vi "AddPerformancePropertiesToWaveform.vi"(6 "Waveform":waveform(sgl), 8 "error in (no error)":errorcluster, 9 "Channel":string, 10 "Group":string, 11 "Tdms Ref":refnum<k34>) -> (0 "error out":errorcluster, 1 "Channel out":string, 2 "Group out":string, 3 "Tdms Ref out":refnum<k34>)   [LabVIEW 2017, in "DataExplorerSupport.lvlib"]
uses:
  <vilib>/addons/InsightCM/Utilities/DataExplorerSupport/DataExplorerSupport.lvlib
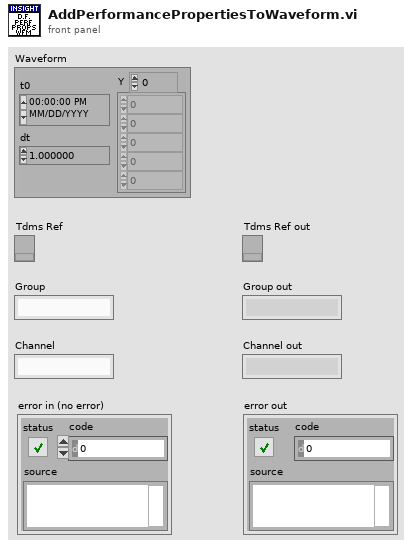
[diagram p1: front panel]
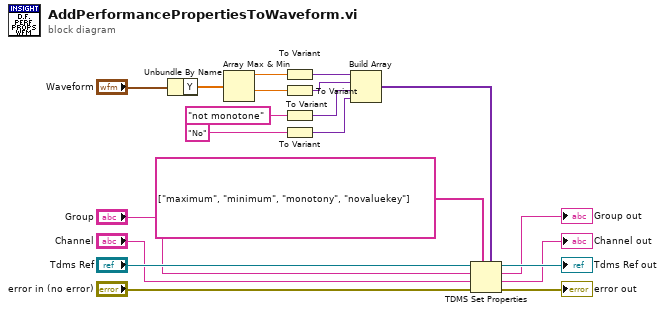
[diagram p0: block diagram]
diagram:
  n1 = Unbundle By Name("Waveform") -> ("Y"=w11:sgl[])
  n2 = Array Max & Min(array=w11) -> (max value=w9:sgl, min value=w7:sgl)  [unwired: 2 out]
  n3 = To Variant(anything=w9) -> (Variant=w8:variant)
  n4 = To Variant(anything=w7) -> (Variant=w6:variant)
  n5 = To Variant(anything="not monotone") -> (Variant=w4:variant)
  n6 = To Variant(anything="No") -> (Variant=w2:variant)
  n7 = Build Array(w8, w6, w4, w2) -> (w1:variant[])
  n8 = TDMS Set Properties(5:w1, 7:string[] ["maximum", "minimum", "monotony", "novaluekey"] ("property names"), 8:"error in (no error)", 9:"Channel", 10:"Group", 11:"Tdms Ref") -> (0:→"error out":errorcluster, 1:→"Channel out":string, 2:→"Group out":string, 3:→"Tdms Ref out":refnum<k34>)
